vi "Update Piece Pixels.vi"(8 "error in (no error)":errorcluster caption="entrée d'erreur (pas d'erreur)", 11 "Game Board en entrée":refnum<class "Game Board.lvclass">) -> (0 "error out":errorcluster caption="sortie d'erreur", 3 "Game Board en sortie":refnum<class "Game Board.lvclass">)   [LabVIEW 2017, in "Game Board.lvclass"]
uses:
  Game Board.lvclass
  Game Board.lvclass/Game Board.ctl
  Piece of Bricks_class/Piece of Bricks.lvclass
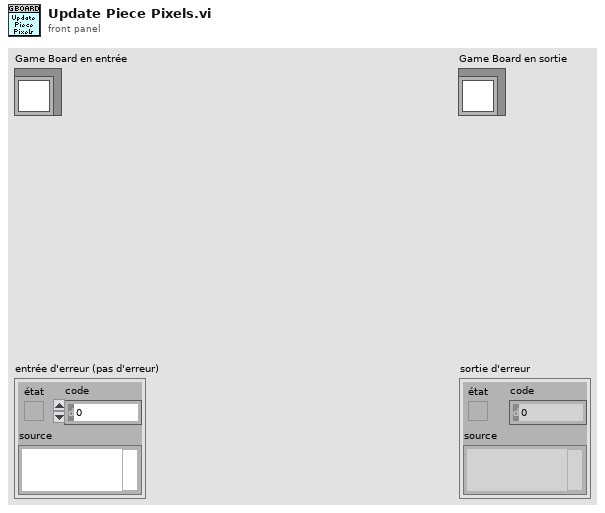
[diagram p1: front panel]
types:
  T1 = typedef "Coordinates.ctl" = cluster{"X":i32, "Y":i32}
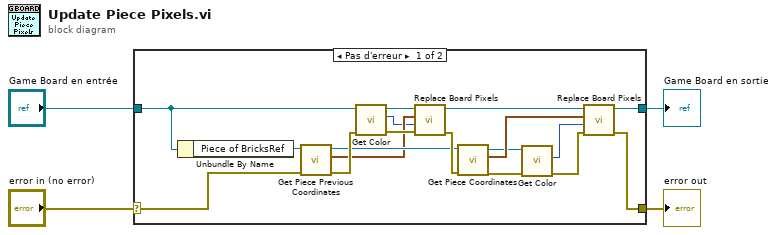
[diagram p0: block diagram]
diagram:
  n1 = case shown="Pas d'erreur" "error in (no error)" {
    selector: "error in (no error)" -> [w10 w24]
    tunnel: [w13 w24] -> w3
    tunnel: [w19 w23] -> w1
    tunnel: "Game Board en entrée" -> [w9 w23]
    frame No Error {
      n2 = Unbundle By Name(w9) -> ("Piece of BricksRef"=w12:refnum<class "Piece of Bricks.lvclass">)
      n3 = call-dynamic "Get Piece Previous Coordinates.vi"("error in (no error)"=w10, "object in"=w12) -> ("error out"=w22:errorcluster, "Piece Previous Coordinates"=w6:T1[], "object out"=w11:refnum<class "Piece of Bricks.lvclass">)  [unwired: 7 in]
      n4 = call-dynamic "Get Color.vi"("error in (no error)"=w22, "object in"=w9) -> ("error out"=w21:errorcluster, "Color"=w5:u32, "object out"=w7:refnum<class "Game Board.lvclass">)  [unwired: 7 in]
      n5 = call-dynamic "Replace Board Pixels.vi"("error in (no error)"=w21, "New pixels color"=w5, "Pixels"=w6, "Game Board en entrée"=w7) -> ("error out"=w20:errorcluster, "Game Board en sortie"=w8:refnum<class "Game Board.lvclass">)  [unwired: 6 in]
      n6 = call-dynamic "Get Piece Coordinates.vi"("error in (no error)"=w20, "object in"=w11) -> ("error out"=w15:errorcluster, "Piece Coordinates"=w18:T1[], "object out"=w17:refnum<class "Piece of Bricks.lvclass">)  [unwired: 7 in]
      n7 = call-dynamic "Get Color.vi"("error in (no error)"=w15, "object in"=w17) -> ("error out"=w14:errorcluster, "Color"=w16:u32)  [unwired: 7 in, 1 out]
      n8 = call-dynamic "Replace Board Pixels.vi"("error in (no error)"=w14, "New pixels color"=w16, "Pixels"=w18, "Game Board en entrée"=w8) -> ("error out"=w13:errorcluster, "Game Board en sortie"=w19:refnum<class "Game Board.lvclass">)  [unwired: 6 in]
    }
    frame Error {
    }
  }
  "error out" <- w3
  "Game Board en sortie" <- w1
